vi "PPSsyncBACKUPVERSION.vi"(5 "Halt":bool, 6 "Advance":bool) -> (0 "Tell Everyone Else to Stop":bool, 1 "PPS":bool, 2 "Timekeeper Locked":bool)   [LabVIEW 2015]
uses:
  <vilib>/FPGAPlugInAG/USRP 294xR; 295xR 120 MSps/niLvFpga_Open_USRP 294xR; 295xR 120 MSps.vi
  <vilib>/rvi/interface/common/dynamic/niFpgaDynamicAddResources.vi
  <vilib>/Utility/error.llb/Error Cluster From Error Code.vi
  <vilib>/rvi/errors/niLvFpgaAdjustHostInterfaceError.vi
  <vilib>/FPGAPlugInAG/Dynamic/niLvFpga_Close_Dynamic.vi
  <vilib>/rvi/interface/nirviOpenFPGA/nirviOpenFPGA.xnode
  FPGA Bitfiles/TimePPS_USRP294xR;295xR1_TimeKeeper_f5VEyXdIdkI.lvbitx
  TimeKeeper.vi
  <vilib>/rvi/interface/nirviReadWriteControl/nirviReadWriteControl.xnode
  <vilib>/rvi/interface/nirviCloseFPGA/nirviCloseFPGA.xnode
  NiFpgaLv.dll
  <vilib>/rvi/interface/Simulation/niFpgaSimulationCallBeginRW.vi
panel:
  out "Epoch Time (ref)":dbl
  out "Offset (ns)":dbl
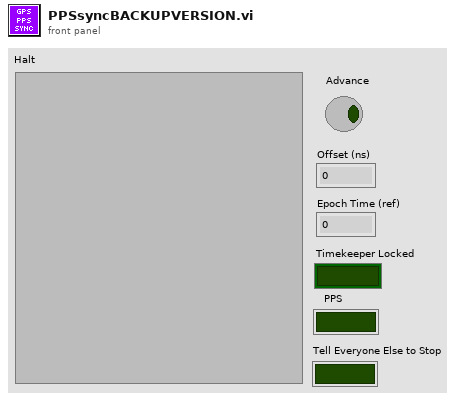
[diagram p1: front panel]
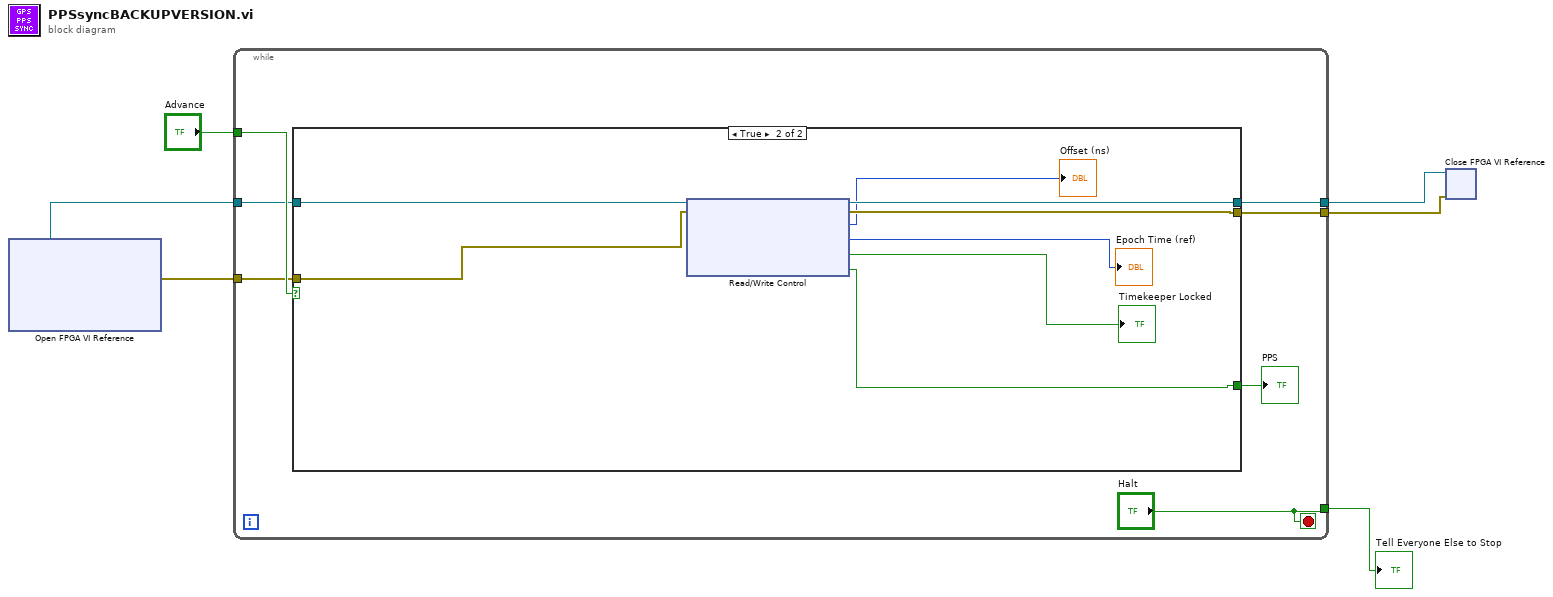
[diagram p0: block diagram]
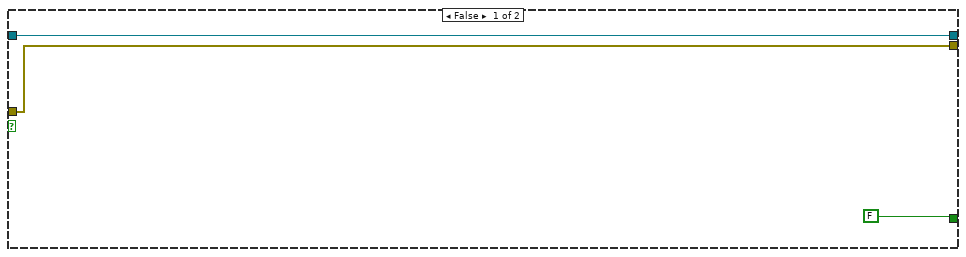
[diagram p2: hidden frame]
diagram:
  n1 = xnode "Open FPGA VI Reference"() -> ("FPGA VI Reference Out"=w2:refnum<k20>, "error out"=w3:errorcluster)  [unwired: 2 in]
  n2 = while {
    tunnel: "Advance" -> [w13]
    tunnel: [w12] -> w5
    tunnel: [w11] -> w4
    tunnel: w3 -> [w10]
    tunnel: w2 -> [w9]
    tunnel: ["Halt"] -> w1
    stop <- "Halt" stop-if-true
    n3 = case shown="True" w13 {
      tunnel: [w16 w24] -> w12
      tunnel: [w15 w23] -> w11
      tunnel: w10 -> [w15 w22]
      tunnel: w9 -> [w16 w21]
      tunnel: [FALSE w17] -> w8
      frame False {
      }
      frame True {
        n4 = xnode "Read/Write Control"("FPGA VI Reference In"=w21, "error in"=w22) -> ("FPGA VI Reference Out"=w24:refnum<k20>, "error out"=w23:errorcluster, "offset from time reference"=→"Offset (ns)":i32, "FPGA Timekeeper time (ns)"=→"Epoch Time (ref)":u64, "FPGA Timekeeper locked"=→"Timekeeper Locked":bool, "PPS"=w17:bool)
      }
    }
    "PPS" <- w8
  }
  "Tell Everyone Else to Stop" <- w1
  n5 = xnode "Close FPGA VI Reference"("FPGA VI Reference In"=w5, "error in"=w4) -> ()  [unwired: 1 out]
